vi "_Axis_SetDec.vi"(8 "Error In":errorcluster, 10 "减速度值":i32, 11 "轴序号":u16) -> (0 "Error Out":errorcluster)   [LabVIEW 2020, in "MT_API.lvlib"]
doc: "MT_API INT32 __stdcall MT_Set_Axis_Position_Dec(WORD AObj,INT32 Value);"
uses:
  MT_API.lvlib
  MT_API_64.dll
panel:
  out "函数返回值":i32
  # "设置轴位置模式下加速度"
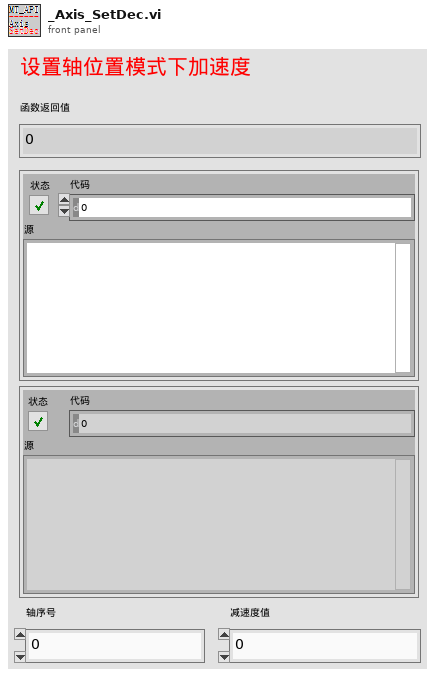
[diagram p1: front panel]
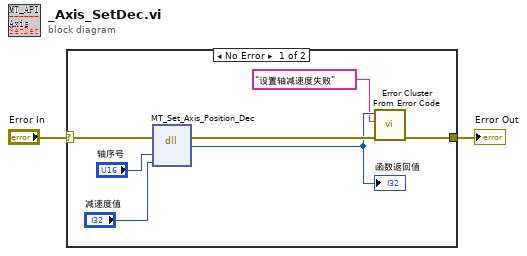
[diagram p0: block diagram]
diagram:
  n1 = case shown="No Error" "Error In" {
    selector: "Error In" -> [w4 w10]
    tunnel: [w3 w10] -> w1
    frame No Error {
      n2 = dll-call lib="D:/Project NJU/lib/MT/MT_API_64.*" fn="MT_Set_Axis_Position_Dec"(error in=w4, "AObj"="轴序号", "Value"="减速度值") -> (error out=w7:errorcluster, "return type"=w6:i32)  [unwired: 4 in, 1 out]
      "函数返回值" <- w6
      n3 = call <vilib>:"Error Cluster From Error Code.vi"("error in (no error)"=w7, "error message (\"\")"="设置轴减速度失败", "error code (0)"=w6) -> ("error out"=w3:errorcluster)  [unwired: 6 in]
    }
    frame Error {
    }
  }
  "Error Out" <- w1
